vi "fgv_counter.vi"(9 "function":T1=enum."Read", 11 "data in":i32) -> (3 "data out":i32)   [LabVIEW 2021]
doc: "本VI是为《我和LabVIEW》一书编写的示例。\n关于本书的介绍请参考网页：\nhttp://ruanqizhen.spaces.live.com/blog/cns!5852D4F797C53FB6!4310.entry"
uses:
  fgv_function.ctl
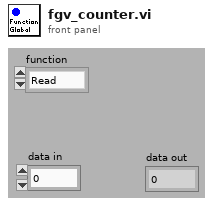
[diagram p1: front panel]
types:
  T1 = typedef "fgv_function.ctl" = enum16{"Reset", "Increase", "Decrease", "Read"}
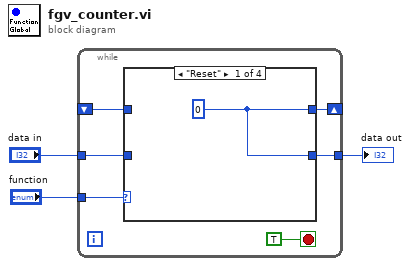
[diagram p0: block diagram]
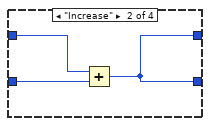
[diagram p2: hidden frame]
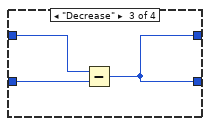
[diagram p3: hidden frame]
diagram:
  n1 = while {
    tunnel: "function" -> [w9]
    tunnel: "data in" -> [w8]
    tunnel: [w7] -> w1
    shift-right: [w5] -> _
    shift-left: _ -> [w6]
    stop <- TRUE stop-if-true
    n2 = case shown="\"Reset\"" w9 {
      tunnel: [w10 w11 w14 w17] -> w7
      tunnel: w6 -> [_ w13 w16 w17]
      tunnel: w8 -> [_ w12 w15 _]
      tunnel: [w10 w11 w14 w17] -> w5
      frame "Reset" {
        w10 = 0
      }
      frame "Increase" {
        n3 = Add(x=w13, y=w12) -> (x+y=w11:i32)
      }
      frame "Decrease" {
        n4 = Subtract(x=w16, y=w15) -> (x-y=w14:i32)
      }
      frame "Read" {
      }
    }
  }
  "data out" <- w1
